vi "Import New Comics.vi"() -> ()   [LabVIEW 2024]
uses:
  TypeDefs/comic--cluster.ctl
  <userlib>/_OpenG.lib/file/file.llb/Strip Path Extension - String__ogtk.vi
  <userlib>/_OpenG.lib/array/array.llb/Sort 1D Array (String)__ogtk.vi
  <userlib>/_OpenG.lib/array/array.llb/openg_array.lvlib
  <userlib>/_OpenG.lib/file/file.llb/openg_file.lvlib
  <vilib>/httpClient/LabVIEWHTTPClient.lvlib
panel:
  out "Available?":bool
  in  "From json":i32(listbox)
  in  "New Comics":path
  out "new issue cover":picture
  out "json issue cover":picture
  out "current issue cover":picture
  in  "Series":i32(listbox)
  in  "New Issues":i32(listbox)
  in  "JSON Issues":i32(listbox)
  in  "Current Issues":i32(listbox)
  in  "Folder":i32(listbox)
  in  "exit":bool
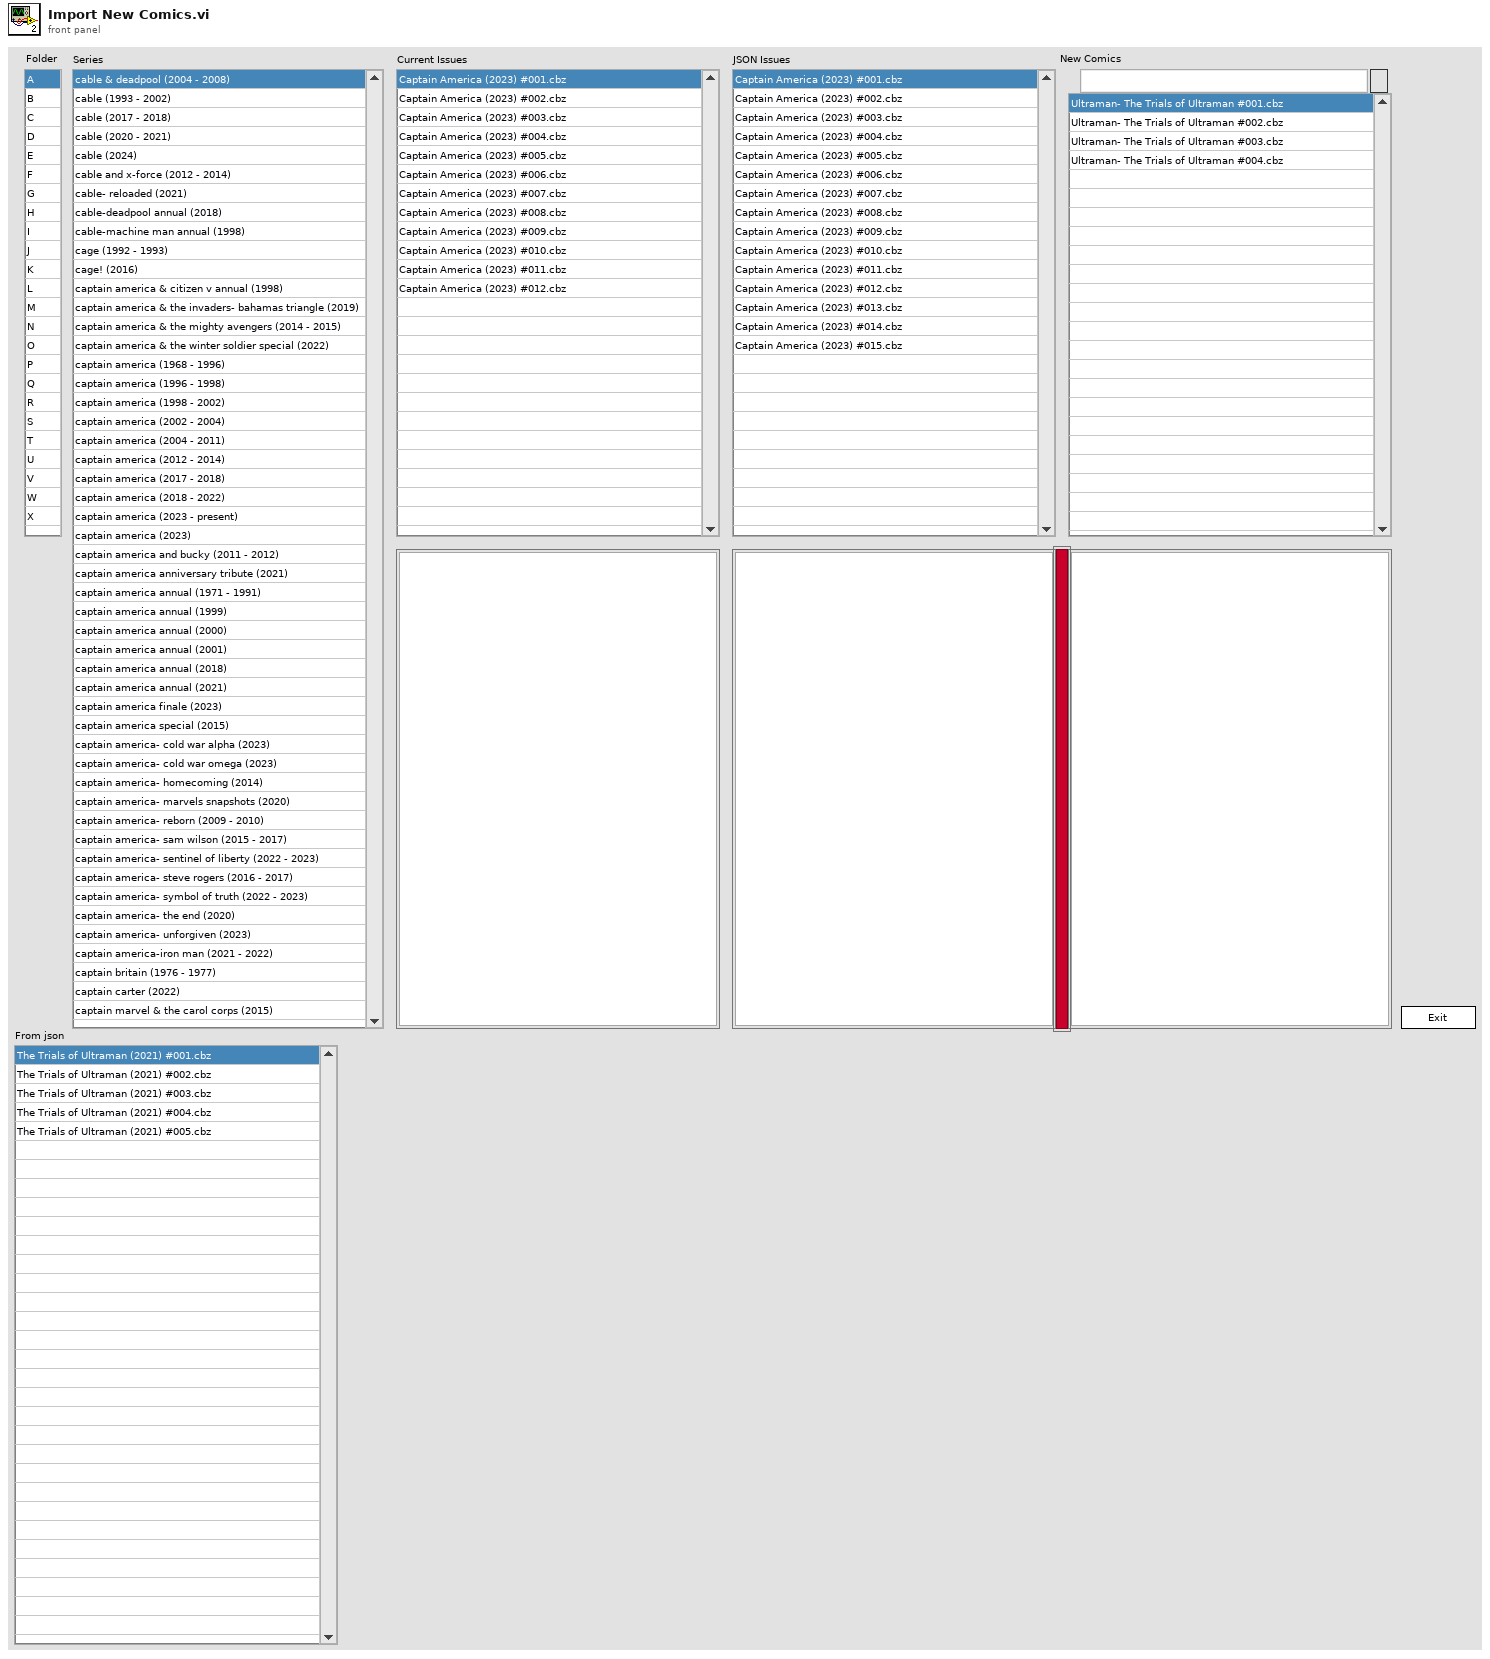
[diagram p1: front panel]
types:
  T1 = enum32{"Invalid", "Standard", "Closed", "Hidden", "Minimized", "Maximized"}
  T2 = enum32{"invalid app kind", "Development System", "Run Time System", "Student Edition", "Embedded LabVIEW", "Evaluation", "Custom"}
  T3 = typedef "comic--cluster.ctl" = cluster{"id":i32, "digitalId":i32, "title":string, "issueNumber":i32, "variantDescription":string, "description":string, "modified":variant, "upc":string, "format":string, "pageCount":i32, "resourceURI":string, "urls":cluster{"type":string, "url":string}[], "series":cluster{"resourceURI":string, "name":string}, "dates":cluster{"type":string, "date":string}[], "prices":cluster{"price":dbl, "type":string}[], "thumbnail":cluster{"path":string, "extension":string}, "images":cluster{"path":string, "extension":string}[], "creators":cluster{"available":i32, "returned":i32, "collectionURI":string, "items":cluster{"resourceURI":string, "name":string, "role":string}[]}, "characters":cluster{"available":i32, "returned":i32, "collectionURI":string, "items":cluster{"resourceURI":string, "name":string}[]}, "stories":cluster{"available":i32, "returned":i32, "collectionURI":string, "items":cluster{"resourceURI":string, "name":string, "type":string}[]}, "events":cluster{"available":i32, "returned":i32, "collectionURI":string, "items":cluster{"resourceURI":string, "name":string}[]}}
  T4 = cluster{"Core":cluster{"Current VI Reference":refnum<vi>, "Close Panel on Exit?":bool}, "repo path":path, "series path":path, "json present":bool, "comic jsons":T3[], "local working folder":path, "web working folder":path, "display web":bool}
  T5 = cluster{"Current VI Reference":refnum<vi>, "Close Panel on Exit?":bool}
  T6 = typedef "imagedata.ctl" = cluster{"image type":i32, "image depth":i32, "image":u8[], "mask":u8[], "colors":u32[], "Rectangle":cluster{"left":i16, "top":i16, "right":i16, "bottom":i16}}
  T7 = typedef "LVBoundsTypeDef.ctl" = cluster{"Width":u32, "Height":u32}
  T8 = typedef "comics.reply--cluster.ctl" = cluster{"code":i32, "status":string, "etag":string, "data":cluster{"offset":i32, "limit":i32, "total":i32, "count":i32, "results":T3[]}}
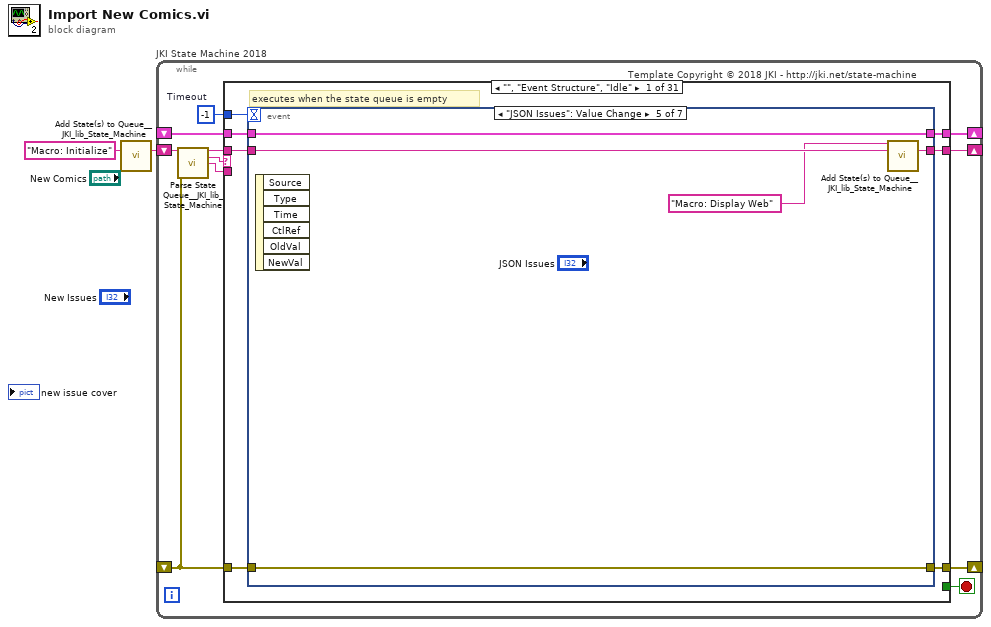
[diagram p0: block diagram]
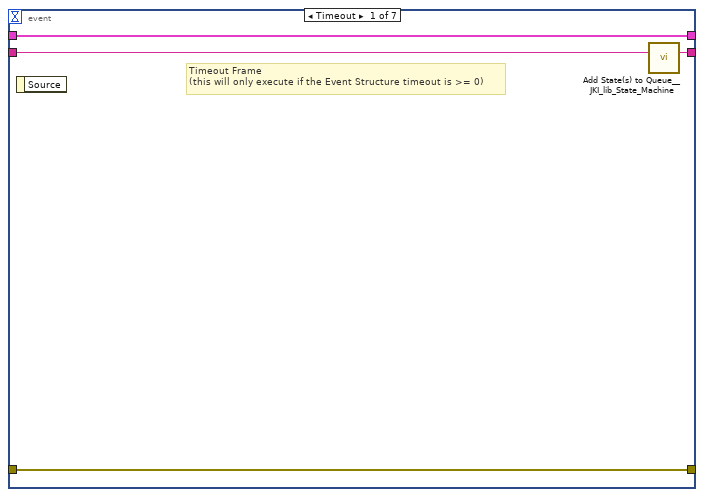
[diagram p2: hidden frame]
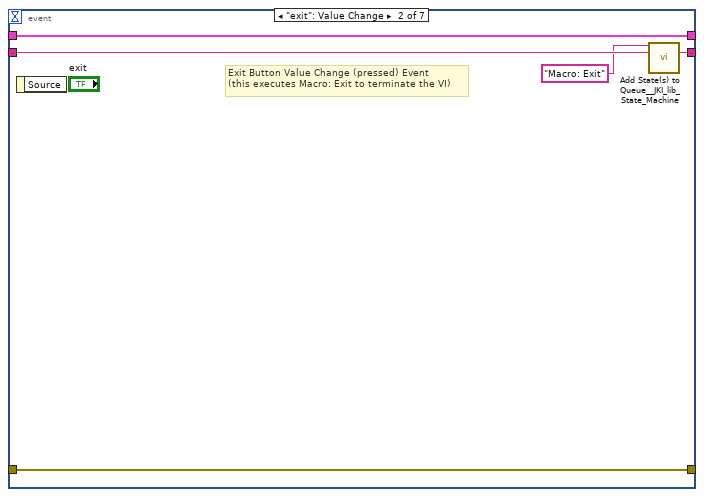
[diagram p3: hidden frame]
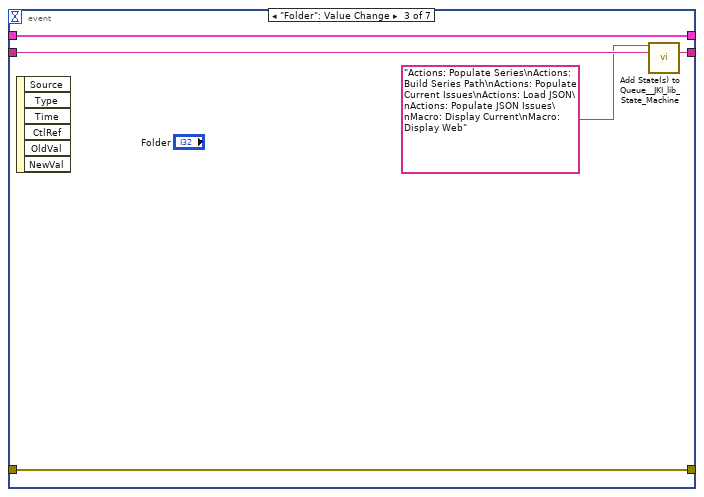
[diagram p4: hidden frame]
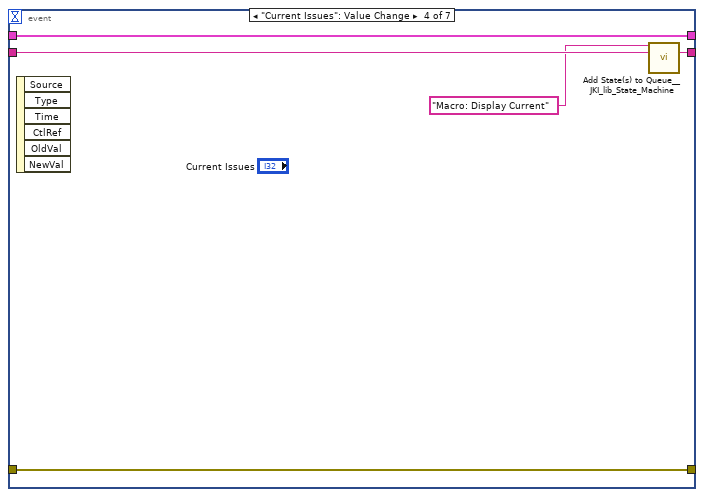
[diagram p5: hidden frame]
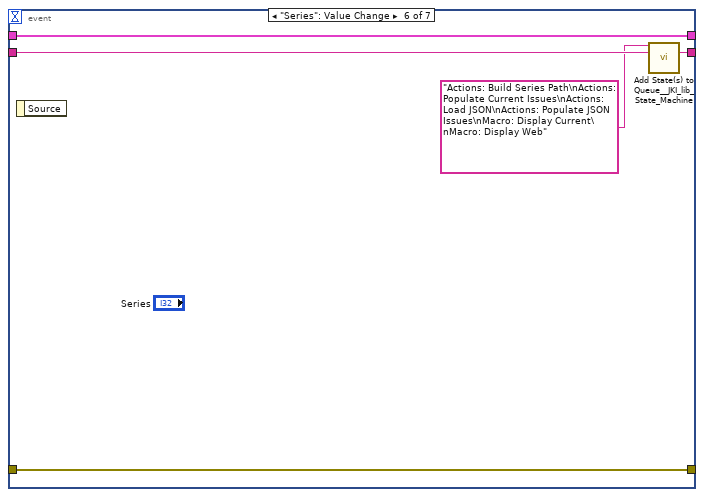
[diagram p6: hidden frame]
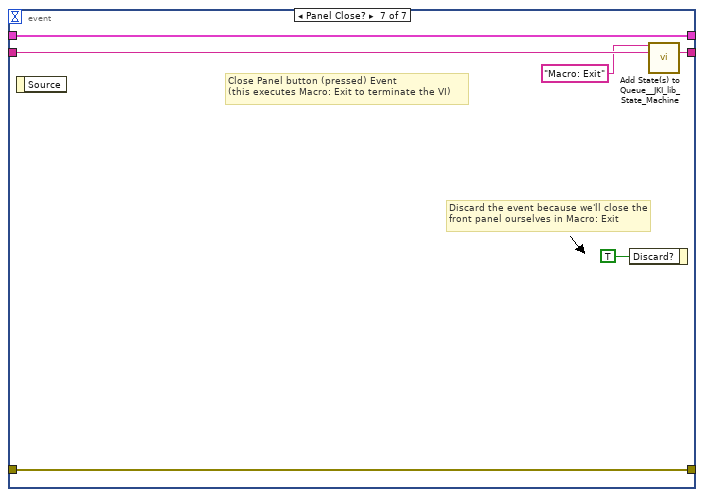
[diagram p7: hidden frame]
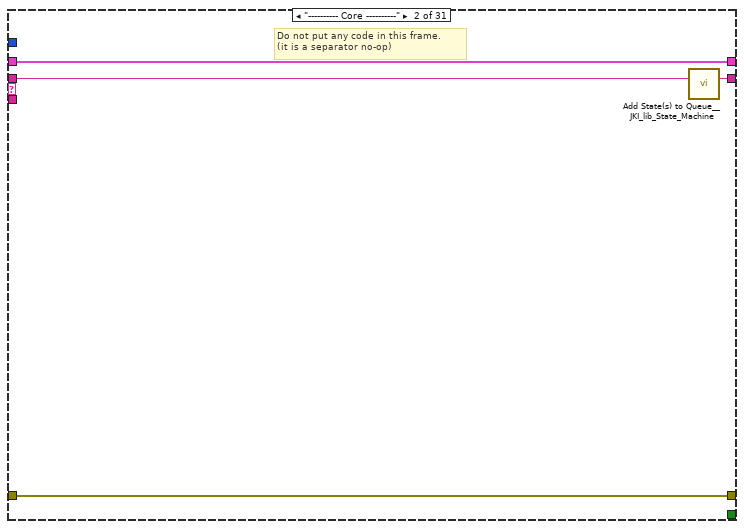
[diagram p8: hidden frame]
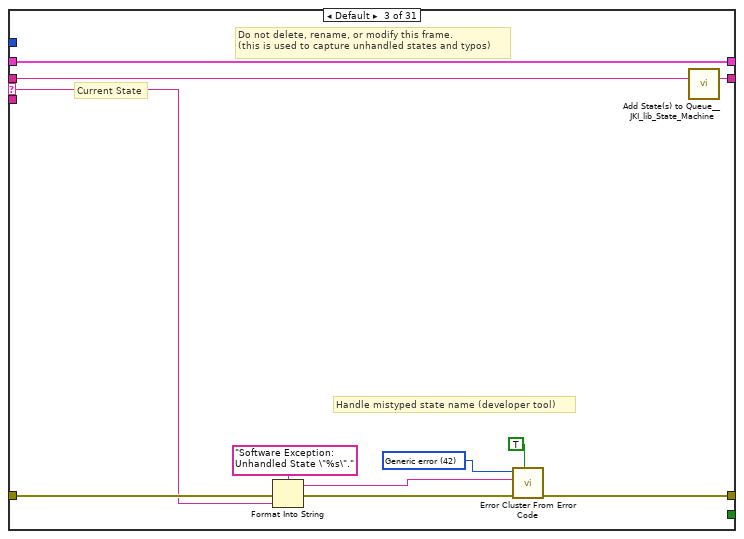
[diagram p9: hidden frame]
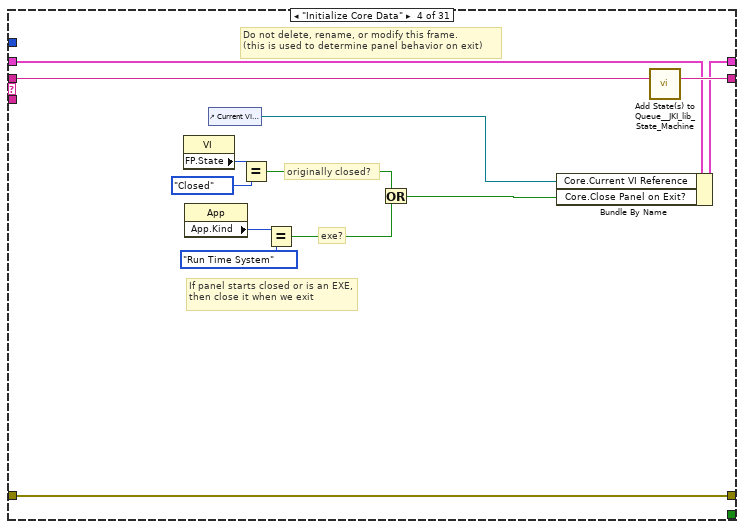
[diagram p10: hidden frame]
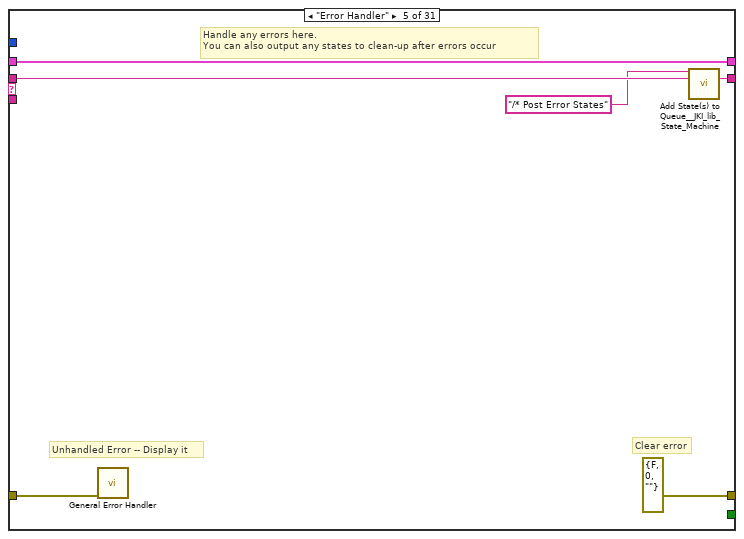
[diagram p11: hidden frame]
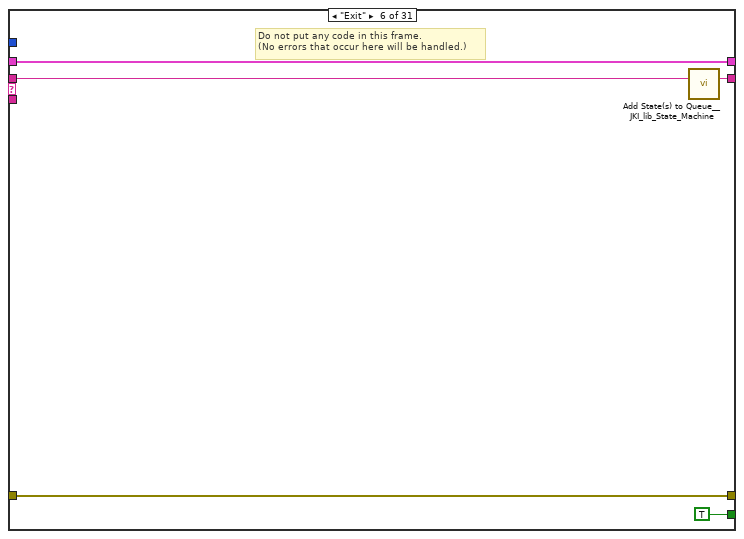
[diagram p12: hidden frame]
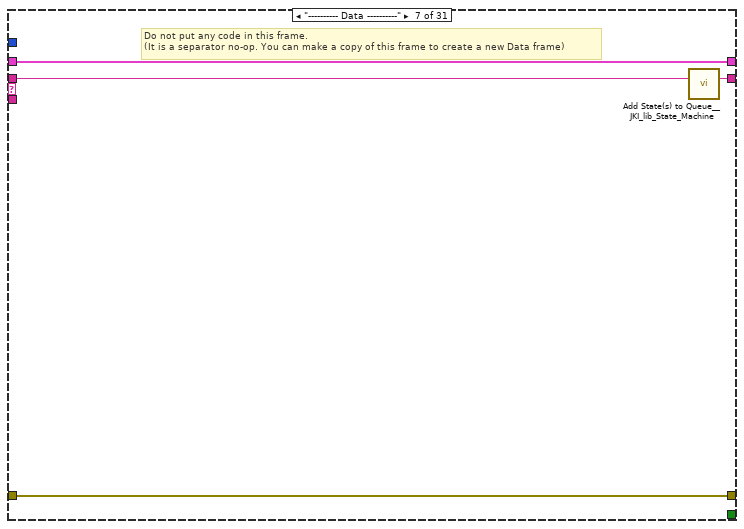
[diagram p13: hidden frame]
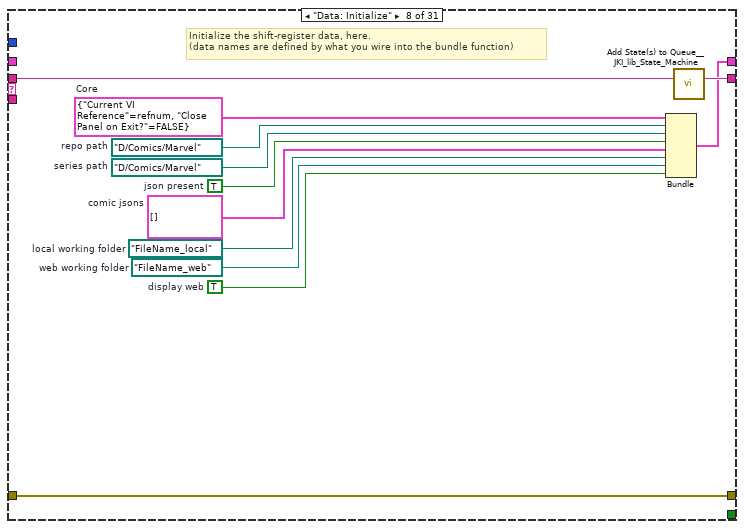
[diagram p14: hidden frame]
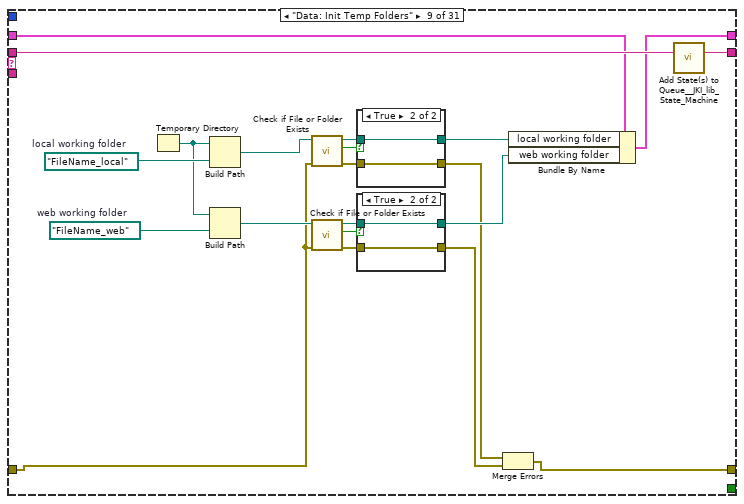
[diagram p15: hidden frame]
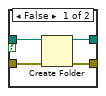
[diagram p16: hidden frame]
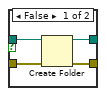
[diagram p17: hidden frame]
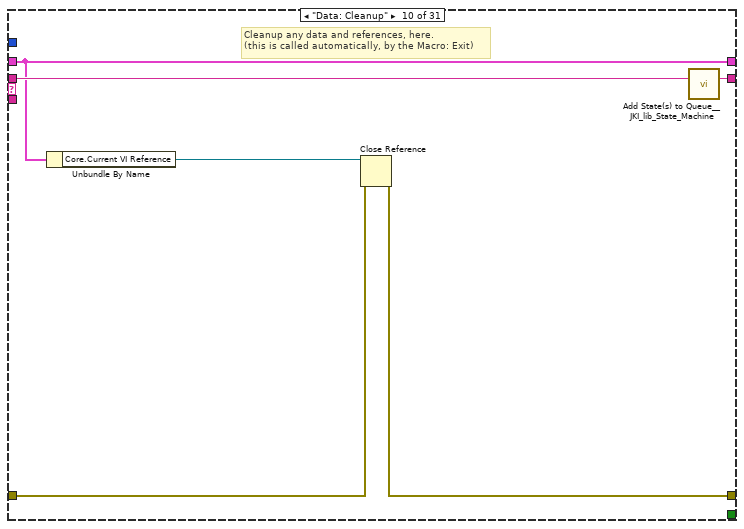
[diagram p18: hidden frame]
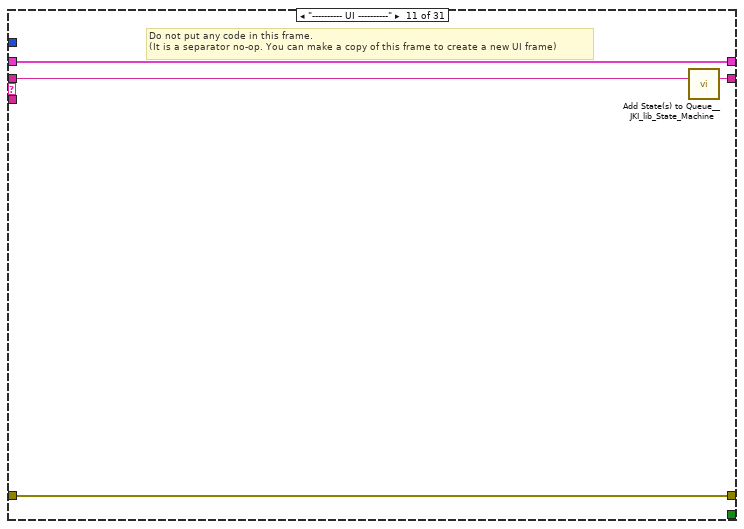
[diagram p19: hidden frame]
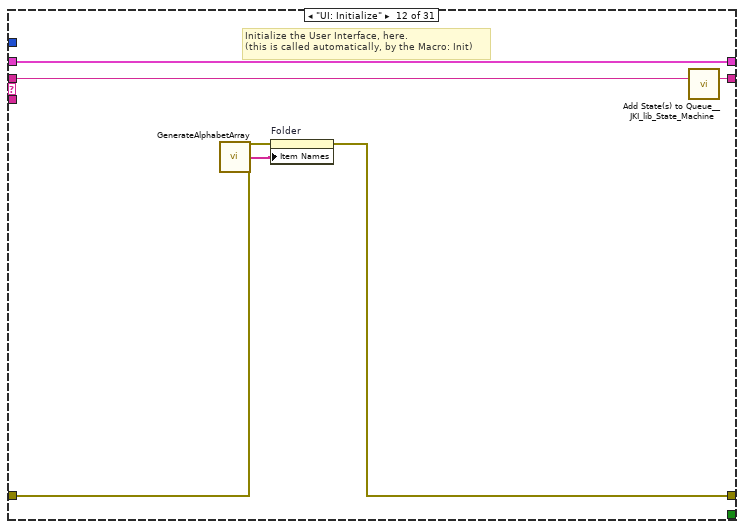
[diagram p20: hidden frame]
diagram:
  n1 = call <vilib>:"Add State(s) to Queue__JKI_lib_State_Machine.vi"("State(s) in (\"\")"="Macro: Initialize") -> ("States Out"=w2:string)  [unwired: 14 in]
  n2 = while "JKI State Machine 2018" {
    shift-right: [w6] -> _
    shift-left: _ -> [w5]
    shift-right: [w9] -> _
    shift-left: _ -> [w3]
    shift-right: [w8] -> _
    shift-left: w2 -> [w10]
    stop <- w7 stop-if-true
    w4 = -1  # Timeout
    # "Template Copyright © 2018 JKI - http://jki.net/state-machine"
    n3 = call <vilib>:"Parse State Queue__JKI_lib_State_Machine.vi"("State Queue"=w10, "Error In (no error)"=w3) -> ("Remaining States"=w12:string, "Current State"=w13:string, "Arguments"=w11:string)  [unwired: 11 in]
    n4 = case shown="\"\", \"Event Structure\", \"Idle\"" w13 {
      selector: w13 -> [_ _ w60 _ _ _ _ _ _ _ _ _ _ _ _ _ _ _ _ _ _ _ _ _ _ _ _ _ _ _ _]
      tunnel: w12 -> [w20 w59 w64 w83 w89 w94 w98 w110 w131 w149 w153 w159 w165 w176 w245 w250 w255 w260 w270 w274 w287 w314 w320 w344 w377 w404 w418 w434 w444 w454 w489]
      tunnel: w11 -> [_ _ _ _ _ _ _ _ _ _ _ _ w160 w170 _ _ _ _ _ _ _ _ _ _ _ _ _ _ _ _ _]
      tunnel: w5 -> [w18 w56 w62 w76 w86 w92 w95 _ w112 w144 w150 w157 w163 w172 w242 w247 w252 w257 w267 w271 w277 w311 w317 w335 w361 w388 w409 w420 w442 w449 w484]
      tunnel: [w17 w57 w66 w80 errorcluster {"status"=FALSE, "code"=0, "source"=""} ("error out") w91 w96 w107 w115 w145 w151 w154 w161 w173 w243 w248 w253 w258 w268 w272 w278 w310 w316 w321 w366 w387 w405 w422 w435 w445 w472] -> w9
      tunnel: w3 -> [w16 w57 w65 w80 w85 w91 w96 w107 w114 w146 w151 w155 w162 w174 w243 w248 w253 w258 w268 w272 w279 w309 w315 w334 w360 w386 w408 w423 w440 w446 w486]
      tunnel: [w19 w58 w63 w82 w88 w93 w97 w109 w130 w148 w152 w158 w164 w175 w244 w249 w254 w259 w269 w273 w286 w313 w319 w343 w376 w403 w417 w433 w443 w453 w488] -> w8
      tunnel: [_ _ _ _ _ TRUE _ _ _ _ _ _ _ _ _ _ _ _ _ _ _ _ _ _ _ _ _ _ _ _ _] -> w7
      tunnel: [w15 w56 w62 w81 w86 w92 w95 w108 w111 w144 w150 w157 w163 w172 w242 w247 w252 w257 w267 w271 w276 w311 w317 w335 w361 w388 w409 w419 w442 w448 w483] -> w6
      tunnel: w4 -> [w14 _ _ _ _ _ _ _ _ _ _ _ _ _ _ _ _ _ _ _ _ _ _ _ _ _ _ _ _ _ _]
      frame "", "Event Structure", "Idle" {
        # "executes when the state queue is empty"
        n5 = event shown="[4] \"JSON Issues\": Value Change" {
          selector: _ -> [_ _ _ _ _ _ _]
          dyn-events: _ -> [_ _ _ _ _ _ _]
          timeout: w14 -> [_ _ _ _ _ _ _]
          tunnel: w20 -> [w24 w29 w34 w39 w44 w49 w55]
          tunnel: [w23 w28 w33 w38 w43 w48 w54] -> w19
          tunnel: w18 -> [w21 w26 w31 w36 w41 w46 w52]
          tunnel: [w22 w27 w32 w37 w42 w45 w53] -> w17
          tunnel: w16 -> [w22 w27 w32 w37 w42 w45 w53]
          tunnel: [w21 w26 w31 w36 w41 w46 w52] -> w15
          event Timeout {
            # "Timeout Frame\n(this will only execute if the Event Structure timeout is >= 0)"
            n6 = event-data() -> ()  [unwired: 1 in, 1 out]
            n7 = call <vilib>:"Add State(s) to Queue__JKI_lib_State_Machine.vi"("State(s) in (\"\")"=w24) -> ("States Out"=w23:string)  [unwired: 14 in]
          }
          event "exit": Value Change {
            # "Exit Button Value Change (pressed) Event\n(this executes Macro: Exit to terminate the VI)"
            n8 = event-data() -> ()  [unwired: 1 in, 1 out]
            n9 = call <vilib>:"Add State(s) to Queue__JKI_lib_State_Machine.vi"("State(s) in Front (\"\")"="Macro: Exit", "State(s) in (\"\")"=w29) -> ("States Out"=w28:string)  [unwired: 13 in]
          }
          event "Folder": Value Change {
            n10 = event-data() -> ()  [unwired: 1 in, 6 out]
            n11 = call <vilib>:"Add State(s) to Queue__JKI_lib_State_Machine.vi"("State(s) in Front (\"\")"="Actions: Populate Series\nActions: Build Series Path\nActions: Populate Current Issues\nActions: Load JSON\nActions: Populate JSON Issues\nMacro: Display Current\nMacro: Display Web", "State(s) in (\"\")"=w34) -> ("States Out"=w33:string)  [unwired: 13 in]
          }
          event "Current Issues": Value Change {
            n12 = event-data() -> ()  [unwired: 1 in, 6 out]
            n13 = call <vilib>:"Add State(s) to Queue__JKI_lib_State_Machine.vi"("State(s) in Front (\"\")"="Macro: Display Current", "State(s) in (\"\")"=w39) -> ("States Out"=w38:string)  [unwired: 13 in]
          }
          event "JSON Issues": Value Change {
            n14 = event-data() -> ()  [unwired: 1 in, 6 out]
            n15 = call <vilib>:"Add State(s) to Queue__JKI_lib_State_Machine.vi"("State(s) in Front (\"\")"="Macro: Display Web", "State(s) in (\"\")"=w44) -> ("States Out"=w43:string)  [unwired: 13 in]
          }
          event "Series": Value Change {
            n16 = event-data() -> ()  [unwired: 1 in, 1 out]
            n17 = call <vilib>:"Add State(s) to Queue__JKI_lib_State_Machine.vi"("State(s) in Front (\"\")"="Actions: Build Series Path\nActions: Populate Current Issues\nActions: Load JSON\nActions: Populate JSON Issues\nMacro: Display Current\nMacro: Display Web", "State(s) in (\"\")"=w49) -> ("States Out"=w48:string)  [unwired: 13 in]
          }
          event Panel Close? {
            # "Discard the event because we'll close the front panel ourselves in Macro: Exit"
            # "Close Panel button (pressed) Event\n(this executes Macro: Exit to terminate the VI)"
            n18 = event-data() -> ()  [unwired: 1 in, 1 out]
            n19 = event-data("Discard?"=TRUE) -> ()  [unwired: 1 in, 1 out]
            n20 = call <vilib>:"Add State(s) to Queue__JKI_lib_State_Machine.vi"("State(s) in Front (\"\")"="Macro: Exit", "State(s) in (\"\")"=w55) -> ("States Out"=w54:string)  [unwired: 13 in]
          }
        }
      }
      frame "---------- Core ----------" {
        # "Do not put any code in this frame.\n(it is a separator no-op)"
        n21 = call <vilib>:"Add State(s) to Queue__JKI_lib_State_Machine.vi"("State(s) in (\"\")"=w59) -> ("States Out"=w58:string)  [unwired: 14 in]
      }
      frame Default {
        w69 = 42 items=["No error", "Argument error", "Memory is full", "Out of zone", "End of file", "File already open", "Generic file I/O error", "File not found", "File permission error", "Disk is full", "Duplicate path", "Too many files open", "System feature not enabled", "Resource file not found", "Cannot add resource", "Resource not found", "Image not found", "Image memory error", "Pen does not exist", "Config type invalid", "Config token not found", "Config parse error", "Config memory error", "Bad external code format", "Bad external code offset", "External code not present", "Null window", "Destroy window error", "Null menu", "Print aborted", "Bad print record", "Print driver error", "Windows error during printing", "Memory error during printing", "Print dialog error", "Generic print error", "Invalid device refnum", "Device not found", "Device parameter error", "Device unit error", "Cannot open device", "Device call aborted", "Generic error", "Cancelled by user", "Object ID too low", "Object ID too high", "Object not in heap", "Unknown heap", "Unknown object (invalid DefProc)", "Unknown object (DefProc not in table)", "Message out of range", "Invalid (null) method", "Unknown message", "Manager call not supported", "Bad address", "Network operation in progress", "Network operation timed out", "Connection is busy", "Network attribute not supported", "Network error", "Address in use", "System out of memory", "Connection aborted", "Connection refused", "Not connected", "Already connected", "Connection closed", "Initialization error (interapplication manager)", "Bad occurrence", "Wait on unbound occurrence handler", "Occurrence queue overflow", "Datalog type conflict", "Unused", "Unrecognized type (interapplication manager)", "Memory corrupt", "Failed to make temporary DLL", "Old CIN version", "Drag socket not found", "Failed to load drop-object", "Failed to register OLE object", "Failed to release OLE object", "Format specifier type mismatch", "Unknown format specifier", "Too few format specifiers", "Too many format specifiers", "Scan failed", "Newer CIN version", "Error converting to variant", "Runtime menu error", "Password tampered", "Variant attribute not found", "Incompatible variant data type", "Event data is not available", "Event Store is not present", "Occurrence is not found", "Event Queue is not created", "Event info is not available", "Refnum passed is NULL", "Error retrieving Class GUID", "Error retrieving CoClass GUID", "Error retrieving TypeLib GUID.", "Bad built application magic bytes.", "Specific driver is different from the specific driver associated with the Logical Name.", "There is no session opened to the class driver.", "Max Error", "MAX - Error with config objects", "MAX - Error loading configuration", "MAX - Group not supported"]
        # "Current State"
        # "Do not delete, rename, or modify this frame.\n(this is used to capture unhandled states and typos)"
        # "Handle mistyped state name (developer tool)"
        n22 = Format Into String(format string="Software Exception: Unhandled State \"%s\"." ("message"), error in=w65, w60) -> (resulting string=w68:string, error out=w67:errorcluster)  [unwired: 1 in]
        n23 = call <vilib>:"Error Cluster From Error Code.vi"("show call chain? (False)"=TRUE, "error in (no error)"=w67, "error message (\"\")"=w68, "error code (0)"=w69) -> ("error out"=w66:errorcluster)  [unwired: 5 in]
        n24 = call <vilib>:"Add State(s) to Queue__JKI_lib_State_Machine.vi"("State(s) in (\"\")"=w64) -> ("States Out"=w63:string)  [unwired: 14 in]
      }
      frame "Initialize Core Data" {
        # "Do not delete, rename, or modify this frame.\n(this is used to determine panel behavior on exit)"
        # "originally closed?"
        # "exe?"
        # "If panel starts closed or is an EXE, then close it when we exit"
        n25 = property class="VI"() -> ("FP.State"=w73:T1)  [unwired: 2 in, 2 out]
        n26 = property class="App"() -> ("App.Kind"=w79:T2)  [unwired: 2 in, 2 out]
        n27 = control-ref of="Current VI Reference"() -> (w74:refnum<vi>)
        n28 = Equal?(x=w73, y=T1."Closed" ("Front Panel Window:State")) -> (x = y?=w71:bool)
        n29 = Equal?(x=w79, y=T2."Run Time System" ("Application:Kind")) -> (x = y?=w77:bool)
        n30 = Or(x=w71, y=w77) -> (x .or. y?=w75:bool)
        n31 = Bundle By Name(cluster=w76, "Core.Current VI Reference"=w74, "Core.Close Panel on Exit?"=w75) -> (w81:T4)
        n32 = call <vilib>:"Add State(s) to Queue__JKI_lib_State_Machine.vi"("State(s) in (\"\")"=w83) -> ("States Out"=w82:string)  [unwired: 14 in]
      }
      frame "Error Handler" {
        # "Unhandled Error -- Display it"
        # "Handle any errors here.\nYou can also output any states to clean-up after errors occur"
        # "Clear error"
        n33 = call <vilib>:"General Error Handler.vi"("error in (no error)"=w85) -> ()  [unwired: 10 in, 5 out]
        n34 = call <vilib>:"Add State(s) to Queue__JKI_lib_State_Machine.vi"("State(s) in Front (\"\")"="/* Post Error States", "State(s) in (\"\")"=w89) -> ("States Out"=w88:string)  [unwired: 13 in]
      }
      frame "Exit" {
        # "Do not put any code in this frame.\n(No errors that occur here will be handled.)"
        n35 = call <vilib>:"Add State(s) to Queue__JKI_lib_State_Machine.vi"("State(s) in (\"\")"=w94) -> ("States Out"=w93:string)  [unwired: 14 in]
      }
      frame "---------- Data ----------" {
        # "Do not put any code in this frame.\n(It is a separator no-op. You can make a copy of this frame to create a new Data frame)"
        n36 = call <vilib>:"Add State(s) to Queue__JKI_lib_State_Machine.vi"("State(s) in (\"\")"=w98) -> ("States Out"=w97:string)  [unwired: 14 in]
      }
      frame "Data: Initialize" {
        w99 = TRUE  # display web
        w100 = path "FileName_web"  # web working folder
        w101 = path "FileName_local"  # local working folder
        w102 = T3[] []  # comic jsons
        w103 = TRUE  # json present
        w104 = path "D:/Comics/Marvel"  # series path
        w105 = T5 {"Current VI Reference"=refnum, "Close Panel on Exit?"=FALSE}  # Core
        w106 = path "D:/Comics/Marvel"  # repo path
        # "Initialize the shift-register data, here.\n(data names are defined by what you wire into the bundle function)"
        n37 = Bundle("Core"=w105, "repo path"=w106, "series path"=w104, "json present"=w103, "comic jsons"=w102, "local working folder"=w101, "web working folder"=w100, "display web"=w99) -> (w108:T4)  [unwired: 1 in]
        n38 = call <vilib>:"Add State(s) to Queue__JKI_lib_State_Machine.vi"("State(s) in (\"\")"=w110) -> ("States Out"=w109:string)  [unwired: 14 in]
      }
      frame "Data: Init Temp Folders" {
        w128 = path "FileName_web"  # web working folder
        w129 = path "FileName_local"  # local working folder
        n39 = Temporary Directory() -> (w127:path)
        n40 = Build Path(base path=w127, name or relative path=w129) -> (appended path=w118:path)
        n41 = Build Path(base path=w127, name or relative path=w128) -> (appended path=w126:path)
        n42 = call <vilib>:"Check if File or Folder Exists.vi"("error in (no error)"=w114, "path"=w118) -> ("error out"=w121:errorcluster, "file or folder exists?"=w119:bool, "dup path"=w120:path)  [unwired: 7 in]
        n43 = call <vilib>:"Check if File or Folder Exists.vi"("error in (no error)"=w114, "path"=w126) -> ("error out"=w123:errorcluster, "file or folder exists?"=w125:bool, "dup path"=w124:path)  [unwired: 7 in]
        n44 = case shown="True" w119 {
          tunnel: w120 -> [w135 w137]
          tunnel: w121 -> [w134 w136]
          tunnel: [w133 w137] -> w117
          tunnel: [w132 w136] -> w116
          frame False {
            n45 = Create Folder(path (use dialog)=w135, error in=w134) -> (created path=w133:path, error out=w132:errorcluster)  [unwired: 1 in, 1 out]
          }
          frame True {
          }
        }
        n46 = case shown="True" w125 {
          tunnel: w124 -> [w141 w143]
          tunnel: w123 -> [w140 w142]
          tunnel: [w139 w143] -> w122
          tunnel: [w138 w142] -> w113
          frame False {
            n47 = Create Folder(path (use dialog)=w141, error in=w140) -> (created path=w139:path, error out=w138:errorcluster)  [unwired: 1 in, 1 out]
          }
          frame True {
          }
        }
        n48 = Merge Errors(w116, w113) -> (w115:errorcluster)
        n49 = Bundle By Name(cluster=w112, "local working folder"=w117, "web working folder"=w122) -> (w111:T4)
        n50 = call <vilib>:"Add State(s) to Queue__JKI_lib_State_Machine.vi"("State(s) in (\"\")"=w131) -> ("States Out"=w130:string)  [unwired: 14 in]
      }
      frame "Data: Cleanup" {
        # "Cleanup any data and references, here.\n(this is called automatically, by the Macro: Exit)"
        n51 = Unbundle By Name(w144) -> ("Core.Current VI Reference"=w147:refnum<vi>)
        n52 = Close Reference(reference=w147, error in (no error)=w146) -> (error out=w145:errorcluster)
        n53 = call <vilib>:"Add State(s) to Queue__JKI_lib_State_Machine.vi"("State(s) in (\"\")"=w149) -> ("States Out"=w148:string)  [unwired: 14 in]
      }
      frame "---------- UI ----------" {
        # "Do not put any code in this frame.\n(It is a separator no-op. You can make a copy of this frame to create a new UI frame)"
        n54 = call <vilib>:"Add State(s) to Queue__JKI_lib_State_Machine.vi"("State(s) in (\"\")"=w153) -> ("States Out"=w152:string)  [unwired: 14 in]
      }
      frame "UI: Initialize" {
        # "Initialize the User Interface, here.\n(this is called automatically, by the Macro: Init)"
        n55 = call "GenerateAlphabetArray.vi"() -> ("Array"=w156:string[])
        n56 = property on="Folder" class="LstBox (strict)"(error in=w155, "Item Names"=w156) -> (error out=w154:errorcluster)  [unwired: 1 in, 1 out]
        n57 = call <vilib>:"Add State(s) to Queue__JKI_lib_State_Machine.vi"("State(s) in (\"\")"=w159) -> ("States Out"=w158:string)  [unwired: 14 in]
      }
      frame "UI: Cursor Set" {
        # "Argument"
        # "Set and Unset Cursor Busy.\n(Usage: \"UI: Cursor Set >> Busy|Idle\")"
        n58 = case shown="\"Idle\", Default" w160 {
          tunnel: w162 -> [w167 w169]
          tunnel: [w166 w168] -> w161
          frame "Idle", Default {
            n59 = call <vilib>:"Unset Busy.vi"("error in (no error)"=w167) -> ("error out"=w166:errorcluster)  [unwired: 10 in]
          }
          frame "Busy" {
            n60 = call <vilib>:"Set Busy.vi"("error in (no error)"=w169) -> ("error out"=w168:errorcluster)  [unwired: 9 in, 1 out]
          }
        }
        n61 = call <vilib>:"Add State(s) to Queue__JKI_lib_State_Machine.vi"("State(s) in (\"\")"=w165) -> ("States Out"=w164:string)  [unwired: 14 in]
      }
      frame "UI: Front Panel State" {
        # "Argument"
        # "Set Front Panel Open or Closed\n(Usage: \"UI: Front Panel State >> Open|Close\")"
        n62 = Unbundle By Name(w172) -> ("Core.Current VI Reference"=w171:refnum<vi>)
        n63 = case shown="\"Minimize\", \"Minimized\"" w170 {
          tunnel: w174 -> [w182 w197 w208 w221 w234]
          tunnel: [w184 w198 w210 w223 w236] -> w173
          tunnel: w171 -> [w183 w195 w209 w222 w235]
          frame "Open", "Standard", Default {
            w177 = T1."Standard" ("State")
            n64 = property class="VI"(reference=w183, error in=w182) -> (reference out=w180:refnum<vi>, error out=w181:errorcluster, "FP.State"=w179:T1)
            n65 = Not Equal?(x=w179, y=w177) -> (x != y?=w178:bool)
            n66 = case shown="True" w178 {
              tunnel: [w188 w190] -> w184
              tunnel: w181 -> [w187 w190]
              tunnel: w180 -> [w186 _]
              tunnel: w177 -> [w185 _]
              frame True {
                n67 = invoke class="VI" method="FP.Open"(reference=w186, error in=w187, "Activate"=TRUE, "State"=w185) -> (error out=w188:errorcluster)  [unwired: 1 in, 4 out]
              }
              frame False {
              }
            }
          }
          frame "Close", "Closed" {
            n68 = property class="VI"(reference=w195, error in=w197) -> (reference out=w194:refnum<vi>, error out=w196:errorcluster, "FP.State"=w192:T1)
            n69 = Not Equal?(x=w192, y=T1."Closed" ("Front Panel Window:State")) -> (x != y?=w191:bool)
            n70 = case shown="True" w191 {
              tunnel: [w199 w202] -> w198
              tunnel: w196 -> [w199 w201]
              tunnel: w194 -> [_ w200]
              frame False {
              }
              frame True {
                n71 = invoke class="VI" method="FP.Close"(reference=w200, error in=w201) -> (error out=w202:errorcluster)  [unwired: 1 in, 2 out]
              }
            }
          }
          frame "Hidden", "Hide" {
            w203 = T1."Hidden" ("State")
            n72 = property class="VI"(reference=w209, error in=w208) -> (reference out=w206:refnum<vi>, error out=w207:errorcluster, "FP.State"=w205:T1)
            n73 = Not Equal?(x=w205, y=w203) -> (x != y?=w204:bool)
            n74 = case shown="True" w204 {
              tunnel: [w214 w215] -> w210
              tunnel: w207 -> [w213 w215]
              tunnel: w206 -> [w212 _]
              tunnel: w203 -> [w211 _]
              frame True {
                n75 = invoke class="VI" method="FP.Open"(reference=w212, error in=w213, "State"=w211) -> (error out=w214:errorcluster)  [unwired: 2 in, 4 out]
              }
              frame False {
              }
            }
          }
          frame "Minimize", "Minimized" {
            w216 = T1."Minimized" ("State")
            n76 = property class="VI"(reference=w222, error in=w221) -> (reference out=w219:refnum<vi>, error out=w220:errorcluster, "FP.State"=w218:T1)
            n77 = Not Equal?(x=w218, y=w216) -> (x != y?=w217:bool)
            n78 = case shown="True" w217 {
              tunnel: [w227 w228] -> w223
              tunnel: w220 -> [w226 w228]
              tunnel: w219 -> [w225 _]
              tunnel: w216 -> [w224 _]
              frame True {
                n79 = invoke class="VI" method="FP.Open"(reference=w225, error in=w226, "State"=w224) -> (error out=w227:errorcluster)  [unwired: 2 in, 4 out]
              }
              frame False {
              }
            }
          }
          frame "Maximize", "Maximized" {
            w229 = T1."Maximized" ("State")
            n80 = property class="VI"(reference=w235, error in=w234) -> (reference out=w232:refnum<vi>, error out=w233:errorcluster, "FP.State"=w231:T1)
            n81 = Not Equal?(x=w231, y=w229) -> (x != y?=w230:bool)
            n82 = case shown="True" w230 {
              tunnel: [w240 w241] -> w236
              tunnel: w233 -> [w239 w241]
              tunnel: w232 -> [w238 _]
              tunnel: w229 -> [w237 _]
              frame True {
                n83 = invoke class="VI" method="FP.Open"(reference=w238, error in=w239, "State"=w237) -> (error out=w240:errorcluster)  [unwired: 2 in, 4 out]
              }
              frame False {
              }
            }
          }
        }
        n84 = call <vilib>:"Add State(s) to Queue__JKI_lib_State_Machine.vi"("State(s) in (\"\")"=w176) -> ("States Out"=w175:string)  [unwired: 14 in]
      }
      frame "---------- Macro ----------" {
        # "Do not put any code in this frame.\n(It is a separator no-op. You can make a copy of this frame to create a new Macro frame)"
        n85 = call <vilib>:"Add State(s) to Queue__JKI_lib_State_Machine.vi"("State(s) in (\"\")"=w245) -> ("States Out"=w244:string)  [unwired: 14 in]
      }
      frame "Macro: Display Web" {
        # "Do not put any code in this frame.\n(It is a separator no-op. You can make a copy of this frame to create a new Macro frame)"
        n86 = call <vilib>:"Add State(s) to Queue__JKI_lib_State_Machine.vi"("State(s) in Front (\"\")"="Actions: Clean Web Folder\nActions: Download Cover\nActions: Display Web Cover", "State(s) in (\"\")"=w250) -> ("States Out"=w249:string)  [unwired: 13 in]
      }
      frame "Macro: Display Current" {
        n87 = call <vilib>:"Add State(s) to Queue__JKI_lib_State_Machine.vi"("State(s) in Front (\"\")"="Actions: Clean local Folder\nActions: Expand cbz\nActions: Display Local Cover", "State(s) in (\"\")"=w255) -> ("States Out"=w254:string)  [unwired: 13 in]
      }
      frame "Macro: Initialize" {
        w256 = "Data: Initialize\nInitialize Core Data\nUI: Initialize\nUI: Front Panel State >> Open\nData: Init Temp Folders\nActions: Populate Series"  # Data: Initialize Initialize Core Data UI: Initialize UI: Front Panel State >> Open Data: Init Temp Folders Actions: Populate Series
        # "Initialization Macro\n(This is called once, when the VI starts)"
        n88 = call <vilib>:"Add State(s) to Queue__JKI_lib_State_Machine.vi"("State(s) in Front (\"\")"=w256, "State(s) in (\"\")"=w260) -> ("States Out"=w259:string)  [unwired: 13 in]
      }
      frame "Macro: Exit" {
        # "Exit Macro\n(This is called once, when the VI exits)"
        n89 = Unbundle By Name(w267) -> ("Core.Close Panel on Exit?"=w266:bool)
        n90 = Select(t="UI: Front Panel State >> Close", s=w266, f="") -> (s? t:f=w263:string)
        n91 = call <vilib>:"Add State(s) to Queue__JKI_lib_State_Machine.vi"("State(s) in (\"\")"=w263, "State(s) at Back (\"\")"="Data: Cleanup\nExit") -> ("States Out"=w261:string)  [unwired: 13 in]
        n92 = call <vilib>:"Add State(s) to Queue__JKI_lib_State_Machine.vi"("State(s) in Front (\"\")"=w261, "State(s) in (\"\")"=w270) -> ("States Out"=w269:string)  [unwired: 13 in]
      }
      frame "---------- Actions ----------" {
        # "Template Separator\n(You can make a copy of, or modify, this frame)"
        n93 = call <vilib>:"Add State(s) to Queue__JKI_lib_State_Machine.vi"("State(s) in (\"\")"=w274) -> ("States Out"=w273:string)  [unwired: 14 in]
      }
      frame "Actions: Download Cover" {
        n94 = Unbundle By Name(w277) -> ("json present"=w282:bool, "web working folder"=w283:path, "comic jsons"=w285:T3[])
        n95 = local read "From json"() -> (w284:i32)
        n96 = case shown="True" w282 {
          tunnel: w285 -> [_ w308]
          tunnel: w284 -> [_ w307]
          tunnel: w283 -> [_ w301]
          tunnel: w279 -> [w293 w298]
          tunnel: [w293 w297] -> w281
          tunnel: [_ TRUE] -> w280
          frame False {
          }
          frame True {
            n97 = Index Array(array=w308, index=w307) -> (element=w306:T3)
            n98 = Unbundle By Name(w306) -> ("images"=w305:cluster{"path":string, "extension":string}[])
            n99 = Build Path(base path=w301, name or relative path=path "temp.jpg") -> (appended path=w299:path)
            n100 = Index Array(array=w305) -> (element=w304:cluster{"path":string, "extension":string})  [unwired: 1 in]
            n101 = Unbundle By Name(w304) -> ("path"=w303:string, "extension"=w296:string)
            n102 = Concatenate Strings(w303, "." ("string"), w296) -> (w302:string)
            n103 = call <vilib>:"GET.vi"("output file"=w299, "url"=w302, "error in (no error)"=w298) -> ("error out"=w297:errorcluster)  [unwired: 9 in, 3 out]
          }
        }
        n104 = case shown="Error 59" w281 {
          selector: w281 -> [w289 w290 w292]
          tunnel: [w289 w290 w291] -> w278
          tunnel: [w288 _ _] -> w275
          tunnel: w280 -> [w288 _ _]
          frame No Error {
          }
          frame Default {
          }
          frame Error {
            n105 = call <vilib>:"Clear Errors.vi"("error in (no error)"=w292) -> ("error out"=w291:errorcluster)  [unwired: 5 in, 1 out]
          }
        }
        n106 = Bundle By Name(cluster=w277, "display web"=w275) -> (w276:T4)
        n107 = call <vilib>:"Add State(s) to Queue__JKI_lib_State_Machine.vi"("State(s) in (\"\")"=w287) -> ("States Out"=w286:string)  [unwired: 14 in]
      }
      frame "Actions: Clean Web Folder" {
        n108 = Unbundle By Name(w311) -> ("web working folder"=w312:path)
        n109 = call "ClearWorkingDirectory.vi"("error in"=w309, "Working Path"=w312) -> ("error out"=w310:errorcluster)  [unwired: 8 in, 1 out]
        n110 = call <vilib>:"Add State(s) to Queue__JKI_lib_State_Machine.vi"("State(s) in (\"\")"=w314) -> ("States Out"=w313:string)  [unwired: 14 in]
      }
      frame "Actions: Clean local Folder" {
        n111 = Unbundle By Name(w317) -> ("local working folder"=w318:path)
        n112 = call "ClearWorkingDirectory.vi"("error in"=w315, "Working Path"=w318) -> ("error out"=w316:errorcluster)  [unwired: 8 in, 1 out]
        n113 = call <vilib>:"Add State(s) to Queue__JKI_lib_State_Machine.vi"("State(s) in (\"\")"=w320) -> ("States Out"=w319:string)  [unwired: 14 in]
      }
      frame "Actions: Display Local Cover" {
        n114 = Unbundle By Name(w335) -> ("local working folder"=w342:path)
        n115 = List Folder(path=w342, error in=w334) -> (path out=w340:path, filenames=w341:string[], error out=w339:errorcluster)  [unwired: 2 in, 1 out]
        n116 = Index Array(array=w341) -> (element=w337:string)  [unwired: 1 in]
        n117 = Build Path(base path=w340, name or relative path=w337) -> (appended path=w338:path)
        n118 = call-poly <userlib>:"Strip Path Extension__ogtk.vi"("path"=w337) -> ("extension"=w336:string)  [unwired: 1 out]
        n119 = case shown="\"jpeg\", \"jpg\"" w336 {
          tunnel: w339 -> [w345 w350 w355]
          tunnel: [_ w349 w354] -> w333
          tunnel: [_ w348 w353] -> w326
          tunnel: [w345 w347 w352] -> w324
          tunnel: w338 -> [_ w346 w351]
          frame Default {
          }
          frame "jpeg", "jpg" {
            n120 = call <vilib>:"Read JPEG File.vi"("error in (no error)"=w350, "path to JPEG file"=w346) -> ("error out"=w347:errorcluster, "image data"=w348:T6)  [unwired: 7 in, 1 out]
            n121 = call <vilib>:"Draw Flattened Pixmap.vi"("image data"=w348) -> ("new picture"=w349:picture)  [unwired: 8 in]
          }
          frame "png" {
            n122 = call <vilib>:"Read PNG File.vi"("error in (no error)"=w355, "path to PNG file"=w351) -> ("error out"=w352:errorcluster, "image data"=w353:T6)  [unwired: 7 in, 1 out]
            n123 = call <vilib>:"Draw Flattened Pixmap.vi"("image data"=w353) -> ("new picture"=w354:picture)  [unwired: 8 in]
          }
        }
        "current issue cover" <- w333
        n124 = property on="current issue cover" class="Pict"(error in=w324) -> (error out=w323:errorcluster, "Draw Area Size"=w325:T7)  [unwired: 1 in, 1 out]
        n125 = Unbundle By Name(w326) -> ("Rectangle.right"=w330:i16, "Rectangle.bottom"=w329:i16)
        n126 = Unbundle By Name(w325) -> ("Width"=w332:u32, "Height"=w331:u32)
        n127 = Divide(x=w332, y=w330) -> (x/y=w328:dbl)
        n128 = Divide(x=w331, y=w329) -> (x/y=w327:dbl)
        n129 = Max & Min(x=w328, y=w327) -> (min(x,y)=w322:dbl)  [unwired: 1 out]
        n130 = property on="current issue cover" class="Pict"(error in=w323, "ZoomFactor"=w322) -> (error out=w321:errorcluster)  [unwired: 1 in, 1 out]
        n131 = call <vilib>:"Add State(s) to Queue__JKI_lib_State_Machine.vi"("State(s) in (\"\")"=w344) -> ("States Out"=w343:string)  [unwired: 14 in]
      }
      frame "Actions: Display Web Cover" {
        n132 = Unbundle By Name(w361) -> ("web working folder"=w365:path, "json present"=w363:bool, "display web"=w356:bool)
        "Available?" <- w356
        n133 = And(x=w363, y=w356) -> (x .and. y?=w364:bool)
        n134 = case shown="True" w364 {
          tunnel: [_ w384] -> w358
          tunnel: [w378 w383] -> w359
          tunnel: [_ w382] -> w357
          tunnel: w360 -> [w378 w381]
          tunnel: w365 -> [_ w380]
          tunnel: path "temp.jpg" ("name or relative path") -> [_ w379]
          frame False {
          }
          frame True {
            n135 = Build Path(base path=w380, name or relative path=w379) -> (appended path=w385:path)
            n136 = call <vilib>:"Read JPEG File.vi"("error in (no error)"=w381, "path to JPEG file"=w385) -> ("error out"=w383:errorcluster, "image data"=w384:T6)  [unwired: 7 in, 1 out]
            n137 = call <vilib>:"Draw Flattened Pixmap.vi"("image data"=w384) -> ("new picture"=w382:picture)  [unwired: 8 in]
          }
        }
        "json issue cover" <- w357
        n138 = property on="json issue cover" class="Pict"(error in=w359) -> (error out=w368:errorcluster, "Draw Area Size"=w369:T7)  [unwired: 1 in, 1 out]
        n139 = Unbundle By Name(w358) -> ("Rectangle.right"=w373:i16, "Rectangle.bottom"=w372:i16)
        n140 = Unbundle By Name(w369) -> ("Width"=w375:u32, "Height"=w374:u32)
        n141 = Divide(x=w375, y=w373) -> (x/y=w371:dbl)
        n142 = Divide(x=w374, y=w372) -> (x/y=w370:dbl)
        n143 = Max & Min(x=w371, y=w370) -> (min(x,y)=w367:dbl)  [unwired: 1 out]
        n144 = property on="json issue cover" class="Pict"(error in=w368, "ZoomFactor"=w367) -> (error out=w366:errorcluster)  [unwired: 1 in, 1 out]
        n145 = call <vilib>:"Add State(s) to Queue__JKI_lib_State_Machine.vi"("State(s) in (\"\")"=w377) -> ("States Out"=w376:string)  [unwired: 14 in]
      }
      frame "Actions: Expand cbz" {
        n146 = property on="Current Issues" class="LstBox (strict)"(error in=w386) -> (error out=w389:errorcluster, "Item Names"=w391:string[], "Value"=w390:i32)  [unwired: 1 in, 1 out]
        n147 = Unbundle By Name(w388) -> ("series path"=w393:path, "local working folder"=w395:path)
        n148 = Index Array(array=w391, index=w390) -> (element=w394:string)
        n149 = Build Path(base path=w393, name or relative path=w394) -> (appended path=w392:path)
        n150 = call "PathToQuotedString.vi"("Path"=w395) -> ("String"=w398:string)  [unwired: 10 in]
        n151 = call "PathToQuotedString.vi"("Path"=w392) -> ("String"=w397:string)  [unwired: 10 in]
        n152 = Format Into String(format string="%s e %s -o%s -r", error in=w389, "\"C:\\Program Files\\7-Zip\\7z.exe\"" ("input 1"), w397, w398) -> (resulting string=w400:string, error out=w401:errorcluster)  [unwired: 1 in]
        n153 = call <vilib>:"System Exec.vi"("run minimized? (F)"=TRUE, "error in (no error)"=w401, "command line"=w400) -> ("error out"=w387:errorcluster)  [unwired: 5 in, 3 out]
        n154 = call <vilib>:"Add State(s) to Queue__JKI_lib_State_Machine.vi"("State(s) in (\"\")"=w404) -> ("States Out"=w403:string)  [unwired: 14 in]
      }
      frame "Actions: Populate Series" {
        n155 = Unbundle By Name(w409) -> ("repo path"=w413:path)
        n156 = property on="Folder" class="LstBox (strict)"(error in=w408) -> (error out=w407:errorcluster, "Item Names"=w415:string[], "Value"=w416:i32)  [unwired: 1 in, 1 out]
        n157 = Index Array(array=w415, index=w416) -> (element=w414:string)
        n158 = Build Path(base path=w413, name or relative path=w414) -> (appended path=w410:path)
        n159 = List Folder(path=w410, error in=w407) -> (folder names=w411:string[], error out=w406:errorcluster)  [unwired: 2 in, 2 out]
        n160 = property on="Series" class="LstBox (strict)"(error in=w406, "Item Names"=w411, "Value"=0 ("Series")) -> (error out=w405:errorcluster)  [unwired: 1 in, 1 out]
        n161 = call <vilib>:"Add State(s) to Queue__JKI_lib_State_Machine.vi"("State(s) in (\"\")"=w418) -> ("States Out"=w417:string)  [unwired: 14 in]
      }
      frame "Actions: Build Series Path" {
        n162 = property on="Folder" class="LstBox (strict)"(error in=w423) -> (error out=w427:errorcluster, "Item Names"=w431:string[], "Value"=w430:i32)  [unwired: 1 in, 1 out]
        n163 = Unbundle By Name(w420) -> ("repo path"=w429:path)
        n164 = Index Array(array=w431, index=w430) -> (element=w432:string)
        n165 = property on="Series" class="LstBox (strict)"(error in=w427) -> (error out=w422:errorcluster, "Item Names"=w428:string[], "Value"=w421:i32)  [unwired: 1 in, 1 out]
        n166 = Build Path(base path=w429, name or relative path=w432) -> (appended path=w426:path)
        n167 = Index Array(array=w428, index=w421) -> (element=w425:string)
        n168 = Build Path(base path=w426, name or relative path=w425) -> (appended path=w424:path)
        n169 = Bundle By Name(cluster=w420, "series path"=w424) -> (w419:T4)
        n170 = call <vilib>:"Add State(s) to Queue__JKI_lib_State_Machine.vi"("State(s) in (\"\")"=w434) -> ("States Out"=w433:string)  [unwired: 14 in]
      }
      frame "Actions: Populate Current Issues" {
        n171 = Unbundle By Name(w442) -> ("series path"=w441:path)
        n172 = List Folder(path=w441, pattern="*.cbz", error in=w440) -> (filenames=w438:string[], error out=w437:errorcluster)  [unwired: 1 in, 2 out]
        n173 = property on="Current Issues" class="LstBox (strict)"(error in=w437, "Item Names"=w438, "Value"=0 ("Current Issues")) -> (error out=w435:errorcluster)  [unwired: 1 in, 1 out]
        n174 = call <vilib>:"Add State(s) to Queue__JKI_lib_State_Machine.vi"("State(s) in (\"\")"=w444) -> ("States Out"=w443:string)  [unwired: 14 in]
      }
      frame "Actions: Populate JSON Issues" {
        n175 = Unbundle By Name(w449) -> ("comic jsons"=w451:T3[], "json present"=w450:bool)
        n176 = case shown="True" w450 {
          tunnel: [_ w461] -> w447
          tunnel: w451 -> [_ w459]
          tunnel: w449 -> [w455 w458]
          tunnel: [w455 w456] -> w448
          frame False {
          }
          frame True {
            n177 = for {
              tunnel: w459 -> [w471] mode=indexing
              tunnel: [w466] -> w462 mode=indexing
              n178 = Unbundle By Name(w471) -> ("title"=w470:string)
              n179 = call "BufferComicNameNumber.vi"("string in"=w470) -> ("buffered number string"=w469:string)  [unwired: 10 in]
              n180 = Concatenate Strings(w469, ".cbz" ("string")) -> (w467:string)
              n181 = call "remove.invalid.chars.vi"("string in"=w467) -> ("string out"=w466:string)
            }
            n182 = call-poly <userlib>:"Sort Array__ogtk.vi"("Array in"=w462) -> ("Sorted Pointers"=w460:i32[], "Sorted Array out"=w461:string[])  [unwired: 9 in]
            n183 = for {
              tunnel: w460 -> [w464] mode=indexing
              tunnel: w459 -> [w465]
              tunnel: [w463] -> w457 mode=indexing
              n184 = Index Array(array=w465, index=w464) -> (element=w463:T3)
            }
            n185 = Bundle By Name(cluster=w458, "comic jsons"=w457) -> (w456:T4)
          }
        }
        n186 = property on="JSON Issues" class="LstBox (strict)"(error in=w446, "Item Names"=w447, "Value"=0 ("Current Issues")) -> (error out=w445:errorcluster)  [unwired: 1 in, 1 out]
        n187 = call <vilib>:"Add State(s) to Queue__JKI_lib_State_Machine.vi"("State(s) in (\"\")"=w454) -> ("States Out"=w453:string)  [unwired: 14 in]
      }
      frame "Actions: Load JSON" {
        n188 = Unbundle By Name(w484) -> ("series path"=w487:path)
        n189 = List Folder(path=w487, pattern="comics.*.json", error in=w486) -> (path out=w475:path, filenames=w476:string[], error out=w477:errorcluster)  [unwired: 1 in, 1 out]
        n190 = Index Array(array=w476) -> (element=w482:string)  [unwired: 1 in]
        n191 = Build Path(base path=w475, name or relative path=w482) -> (appended path=w480:path)
        n192 = call <vilib>:"Check if File or Folder Exists.vi"("error in (no error)"=w477, "path"=w480) -> ("error out"=w481:errorcluster, "file or folder exists?"=w478:bool, "dup path"=w479:path)  [unwired: 7 in]
        n193 = case shown="True" w478 {
          selector: w478 -> [w490 w492]
          tunnel: [w491 w496] -> w472
          tunnel: [_ w495] -> w473
          tunnel: w481 -> [w491 w494]
          tunnel: w479 -> [_ w493]
          tunnel: [w490 w492] -> w474
          frame False {
          }
          frame True {
            n194 = Read from Text File(file (use dialog)=w493, error in=w494) -> (text=w499:string, error out=w498:errorcluster)  [unwired: 2 in, 2 out]
            n195 = call "parse.comics_reply.vi"("error in"=w498, "string in"=w499) -> ("error out"=w496:errorcluster, "data"=w497:T8)  [unwired: 8 in]
            n196 = Unbundle By Name(w497) -> ("data.results"=w495:T3[])
          }
        }
        n197 = Bundle By Name(cluster=w484, "json present"=w474, "comic jsons"=w473) -> (w483:T4)
        n198 = call <vilib>:"Add State(s) to Queue__JKI_lib_State_Machine.vi"("State(s) in (\"\")"=w489) -> ("States Out"=w488:string)  [unwired: 14 in]
      }
    }
  }
